vi "Test Cryogens.vi"(8 "error in (no error)":errorcluster) -> (0 "error out":errorcluster)   [LabVIEW 2019]
uses:
  lvsrc/Framework/Instrument Types/Cryostat/Instrument.Cryostat.lvclass
  <vilib>/addons/_JKI Toolkits/Caraya/classes/Assert/Assert Error.vi
  <vilib>/addons/_JKI Toolkits/Caraya/classes/Test/Test.lvclass
  <vilib>/addons/_JKI Toolkits/Caraya/classes/Assert/Assert.lvclass
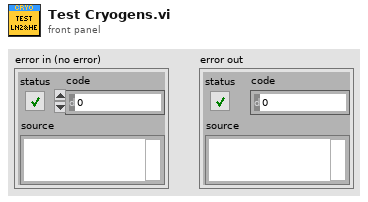
[diagram p1: front panel]
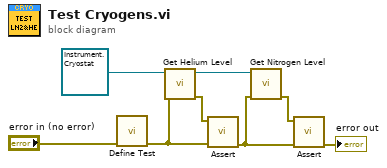
[diagram p0: block diagram]
diagram:
  n1 = call <vilib>:"Define Test.vi"("error in (no error)"="error in (no error)") -> ("error out"=w1:errorcluster)  [unwired: 9 in, 1 out]
  n2 = call-dynamic "Get Helium Level.vi"("error in (no error)"=w1, "Instrument.Cryostat in"=refnum<class "Instrument.Cryostat.lvclass"> refnum) -> ("error out"=w6:errorcluster, "Instrument.Cryostat out"=w5:refnum<class "Instrument.Cryostat.lvclass">)  [unwired: 7 in, 1 out]
  n3 = call-poly <vilib>:"Assert.vi"("error in (no error)"=w1, "Error?"=w6) -> ("error out"=w2:errorcluster)  [unwired: 8 in, 1 out]
  n4 = call-dynamic "Get Nitrogen Level.vi"("error in (no error)"=w2, "Instrument.Cryostat in"=w5) -> ("error out"=w7:errorcluster)  [unwired: 7 in, 2 out]
  n5 = call-poly <vilib>:"Assert.vi"("error in (no error)"=w2, "Error?"=w7) -> ("error out"=→"error out":errorcluster)  [unwired: 8 in, 1 out]
